vi "Calibration_Setting_UI.vi"(5 "Real Position Info":T5, 6 "CamGot?":bool, 7 "Cal Info Image":T1, 8 "error in (no error)":errorcluster, 9 "Cal Status In":bool, 10 "Root Path":path, 11 "Seq":string) -> (0 "error out":errorcluster, 2 "Calibration Done":bool, 3 "CalTemp":T1(plugin-control))   [LabVIEW 2019]
uses:
  <vilib>/vision/Image Controls.llb/IMAQ Image.ctl
  <vilib>/vision/Calibration.llb/Distortion Model.ctl
  <vilib>/vision/Calibration.llb/Distortion Model Types.ctl
  <vilib>/vision/Image Controls.llb/Vision Info Type2.ctl
  Controls/Parameter.ctl
  LLB/Commonly VI/Main Glb.vi
  <vilib>/vision/NI_Vision_Development_Module.lvlib
  LLB/Commonly VI.lvlib
panel:
  in  "Tab Control":enum32{"Page 1", "Page 2"}(tab)
  out "CalTemp 2":T1(plugin-control)
  out "Grid Descriptor 2":T2={"X Step"=1.0, "Y Step"=1.0, "Unit"=enum."Undefined"} {"Y Step" format="%.2f"; "X Step" format="%.2f"}
  in  "CamSelect":u16(ring) caption="相機" items=["cam0"]
  in  "Reset":bool
  in  "Camera Angle":enum32{"Parallel", "Perpendicular"}(radio)
  in  "Relative Position":T4={"Direction"=enum."Negative", "D"=100.0} {"D" min=1.0 step=1.0}
  in  "Reference Points":i32(listbox)
  in  "Use Real Position":bool
  in  "Grid Descriptor":cluster{"X Step":sgl, "Y Step":sgl, "Unit":T3}={"X Step"=10.0, "Y Step"=10.0, "Unit"=enum."Millimeter"}
  in  "Area Min":dbl=100.0
  in  "Area Max":dbl=1000.0
  in  "Run Cal":bool
  in  "CalExit":bool caption="Exit"
  in  "Done":bool
  in  "Snap":bool
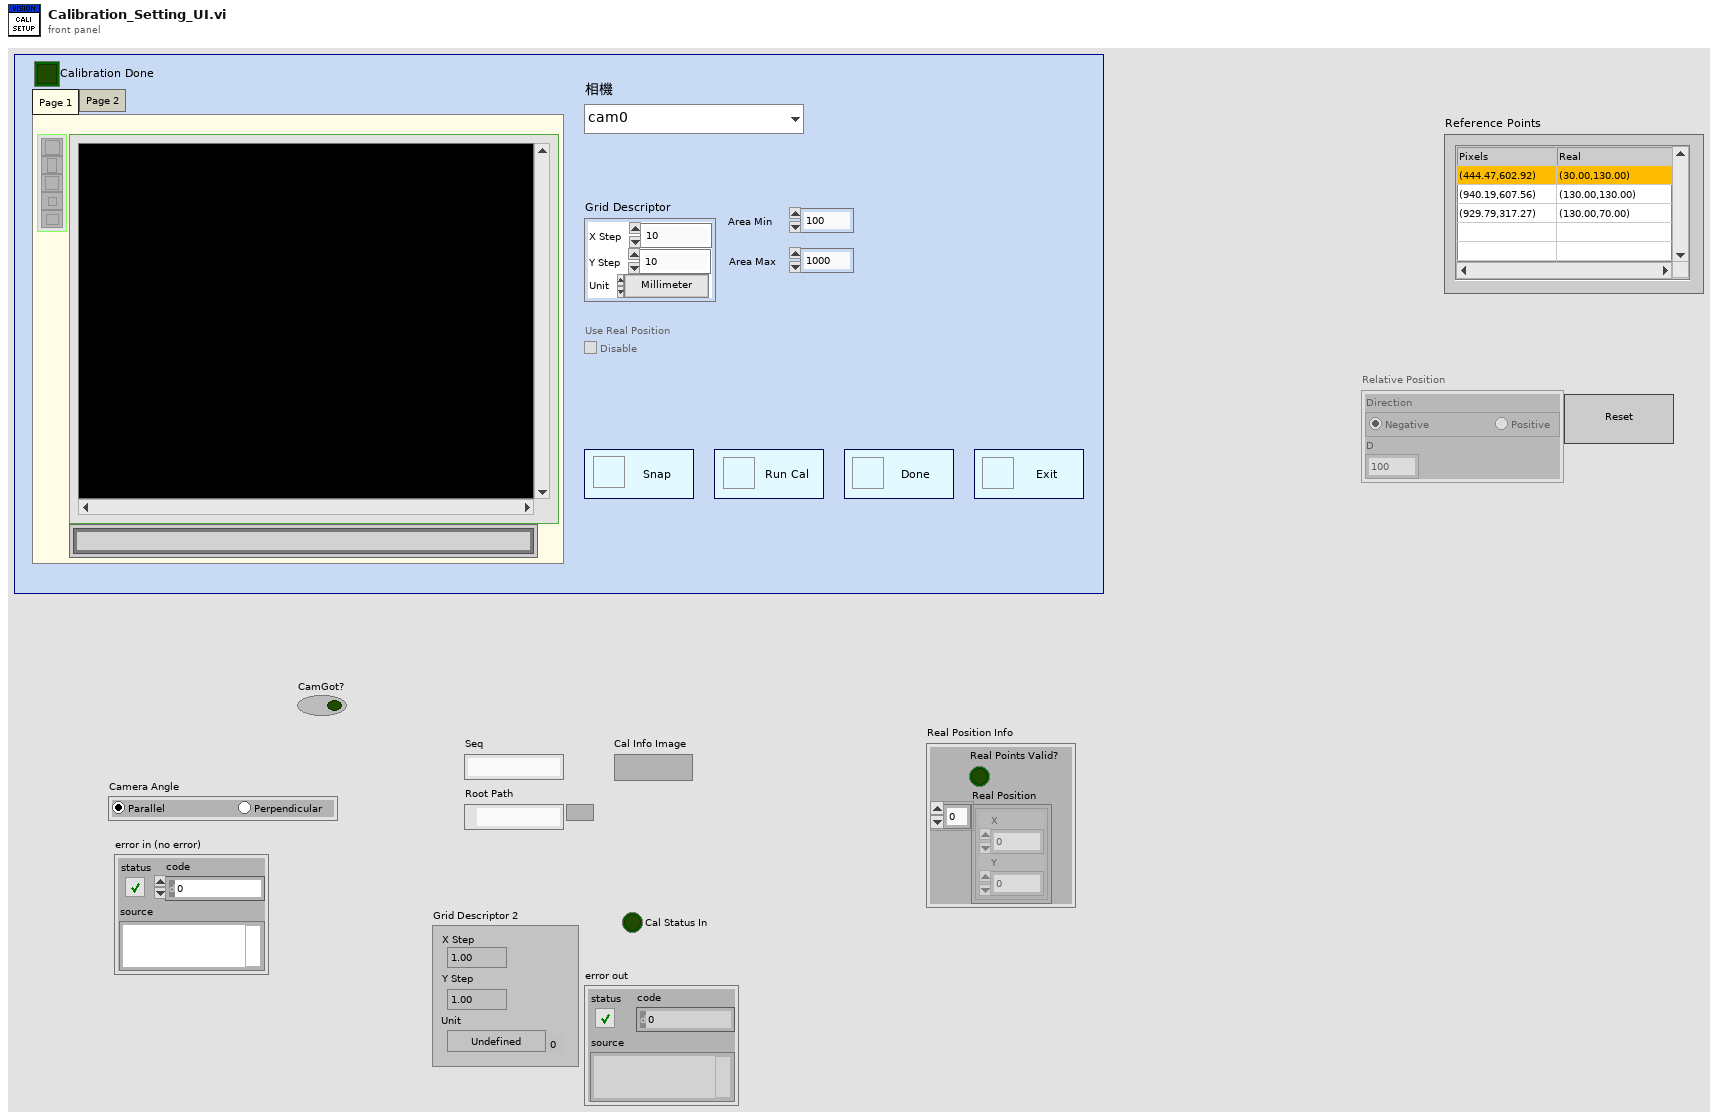
[diagram p1: front panel]
types:
  T1 = typedef "IMAQ Image.ctl" = refnum<image>
  T2 = typedef "Simple Grid Descriptor" = cluster{"X Step":sgl, "Y Step":sgl, "Unit":T3}
  T3 = typedef "Image Unit" = enum32{"Undefined", "Angström", "Micrometer", "Millimeter", "Centimeter", "Meter", "Kilometer", "Microinch", "Inch", "Feet", "Nautical miles", "Standard miles", "Steps"}
  T4 = cluster{"Direction":enum32{"Negative", "Positive"}, "D":dbl}
  T5 = cluster{"Real Points Valid?":bool, "Real Position":cluster{"X":dbl, "Y":dbl}[]}
  T6 = typedef "Image Type" = u32
  T7 = cluster{"Pixel":cluster{"X":dbl, "Y":dbl}[], "Real":cluster{"X":dbl, "Y":dbl}[]}
  T8 = enum16{"Init", "Grab", "Get All", "Close", "Set Camera"}
  T9 = enum8{"Enabled", "Disabled", "Disabled and Grayed Out"}
  T10 = typedef "Distortion Model.ctl" = cluster{"Distortion Model":T11, "Polynomial Model Setup":cluster{"Radial Coefficient":u32, "Tangential Coefficients ":bool}}
  T11 = typedef "Distortion Model Types.ctl" = i32
  T12 = typedef "Parameter.ctl" = enum16{"Initialize", "Write", "Read", "WriteAll", "Save", "Load"}
  T13 = typedef "IMAQdx.ctl" = refnum<k21>
  T14 = cluster{"Global Rectangle":i32[], "Contours":cluster{"Contour Type":u32, "ROI Type":u32, "Points":i32[]}[]}
  T15 = typedef "Calibration Reference Points.ctl" = cluster{"Pixel Coordinates":cluster{"X":dbl, "Y":dbl}[], "Real World Coordinates":cluster{"X":dbl, "Y":dbl}[], "Unit":T3, "Image Size":cluster{"X":u32, "Y":u32}}
  T16 = typedef "ROI Descriptor" = cluster{"Global Rectangle":i32[], "Contours":cluster{"ID":enum32{"External", "Internal"}, "Type":u32, "Coordinates":i32[]}[]}
  T17 = cluster{"Global Rectangle[0]":i32, "Global Rectangle[1]":i32, "Global Rectangle[2]":i32, "Global Rectangle[3]":i32}
  T18 = enum32{"invalid app kind", "Development System", "Run Time System", "Student Edition", "Embedded LabVIEW", "Evaluation", "Custom"}
  T19 = typedef "Vision Info Type2.ctl" = u32
  T20 = cluster{"histogram":u32[], "Minimal Value":sgl, "Maximal Value":sgl, "Starting Value":sgl, "Interval Width":sgl, "Mean Value":sgl, "Standard  Variation":sgl, "Area (pixels)":i32}
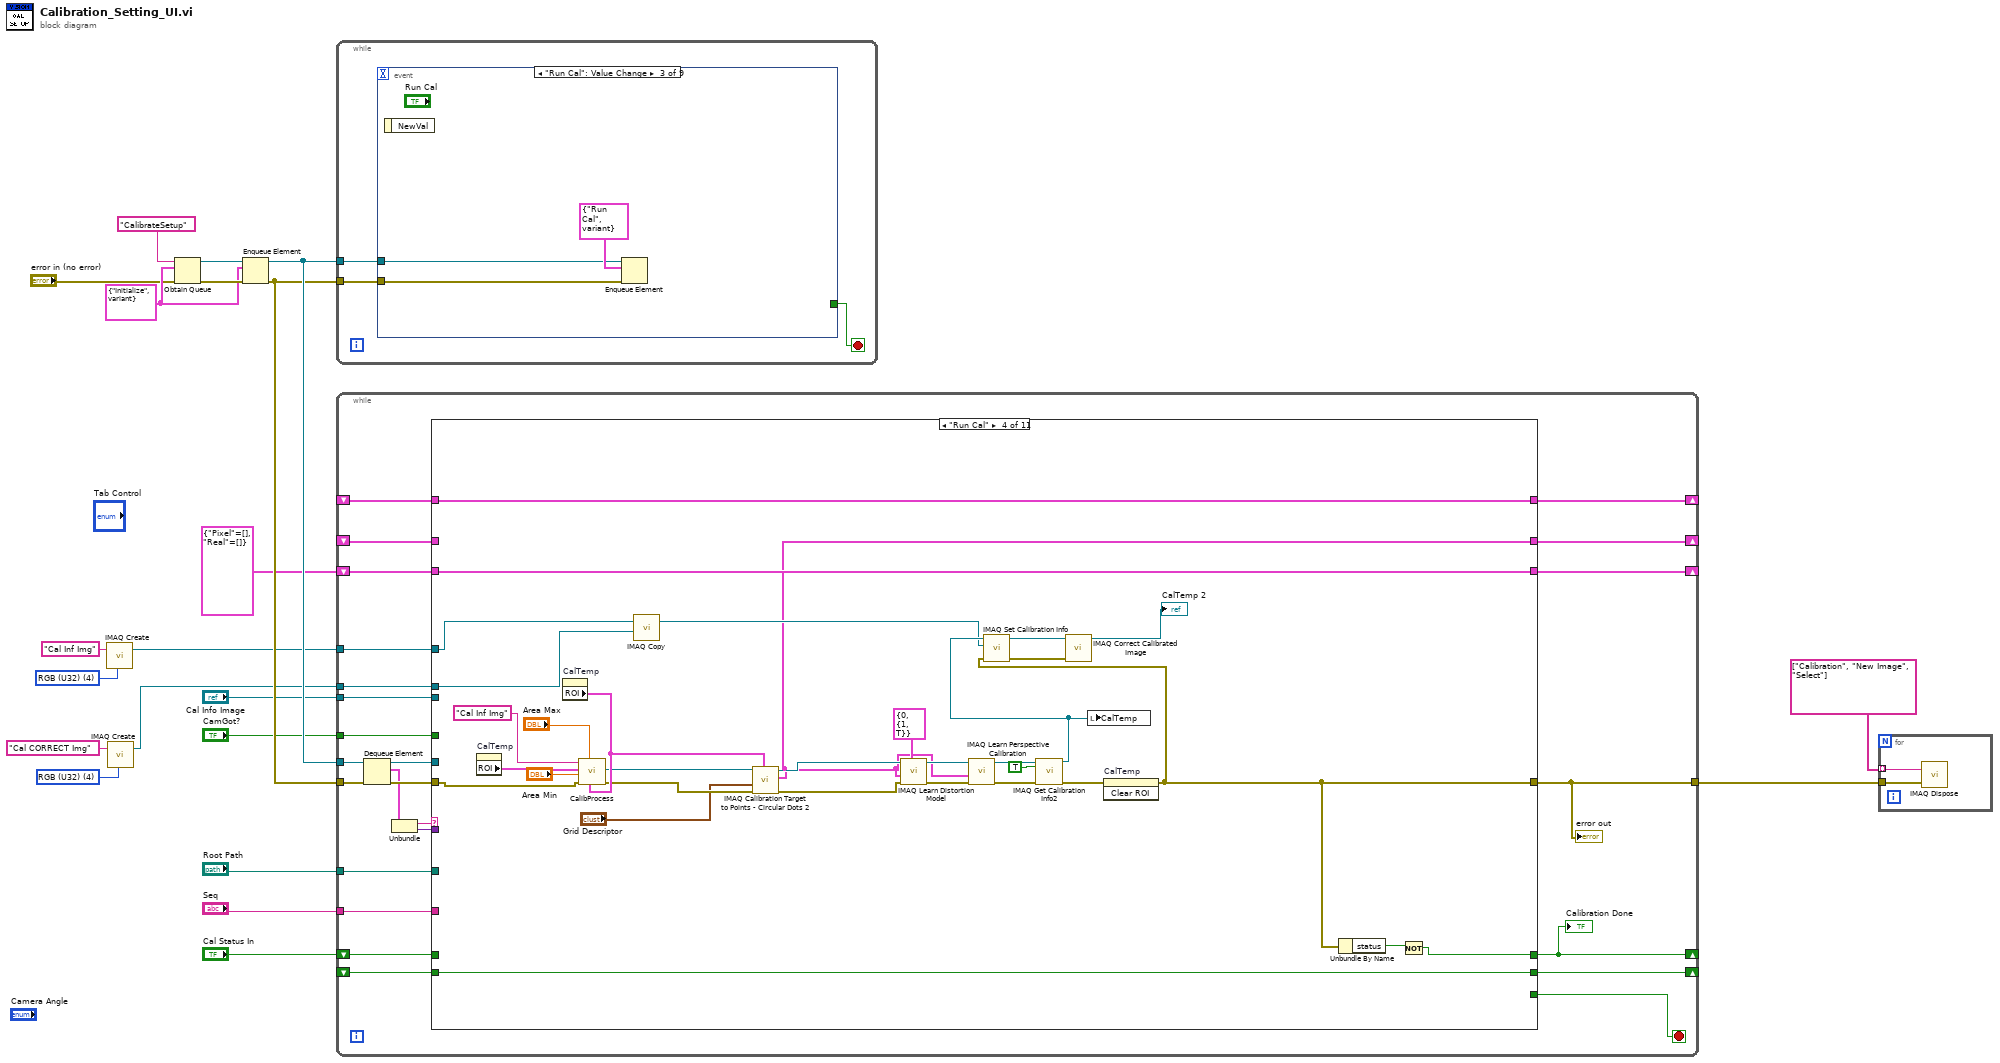
[diagram p0: block diagram]
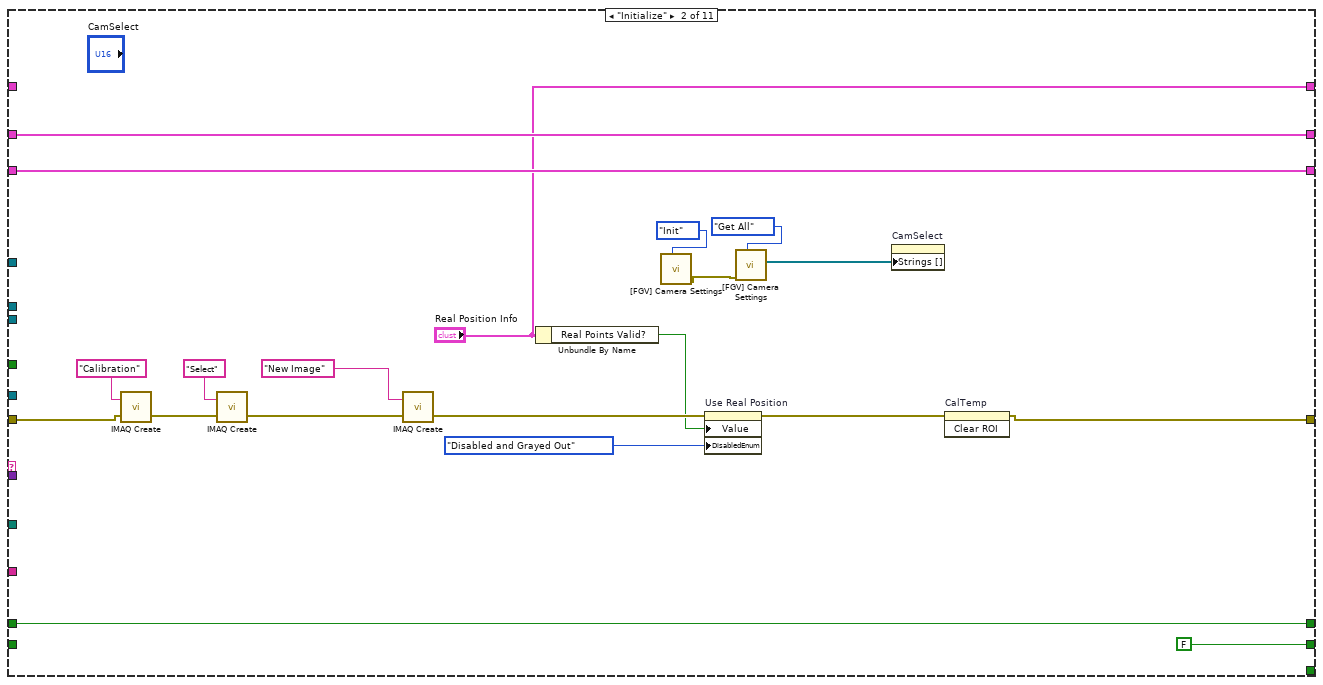
[diagram p3: hidden frame]
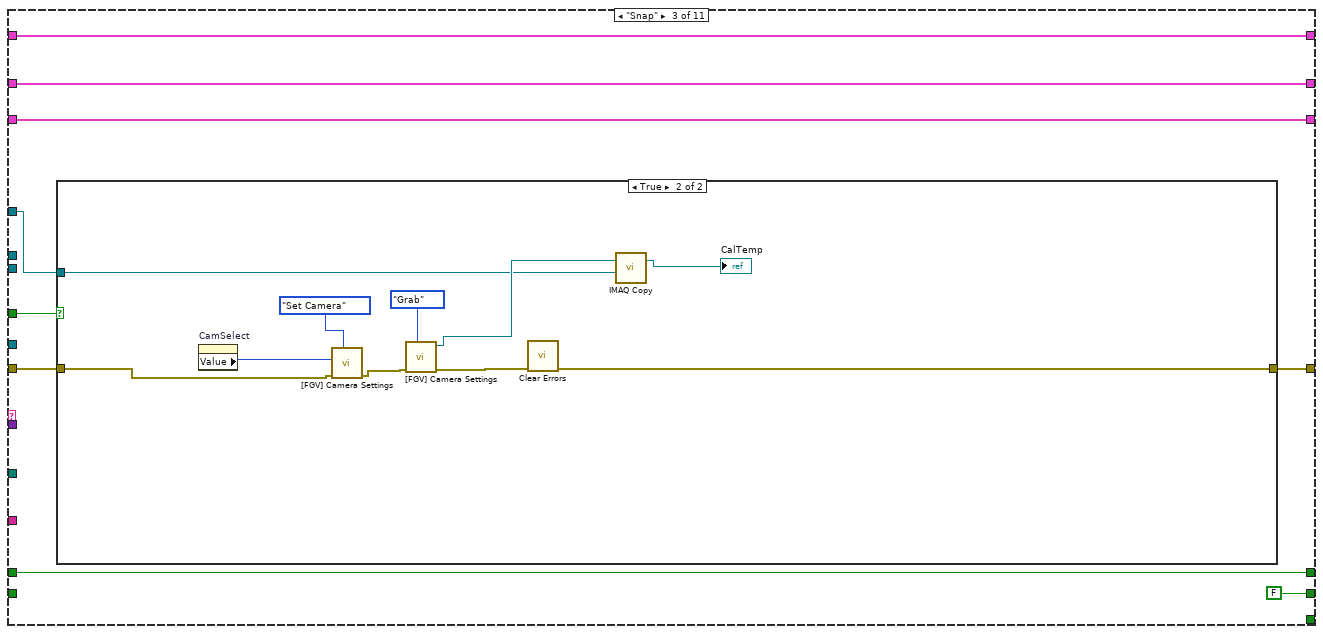
[diagram p4: hidden frame]
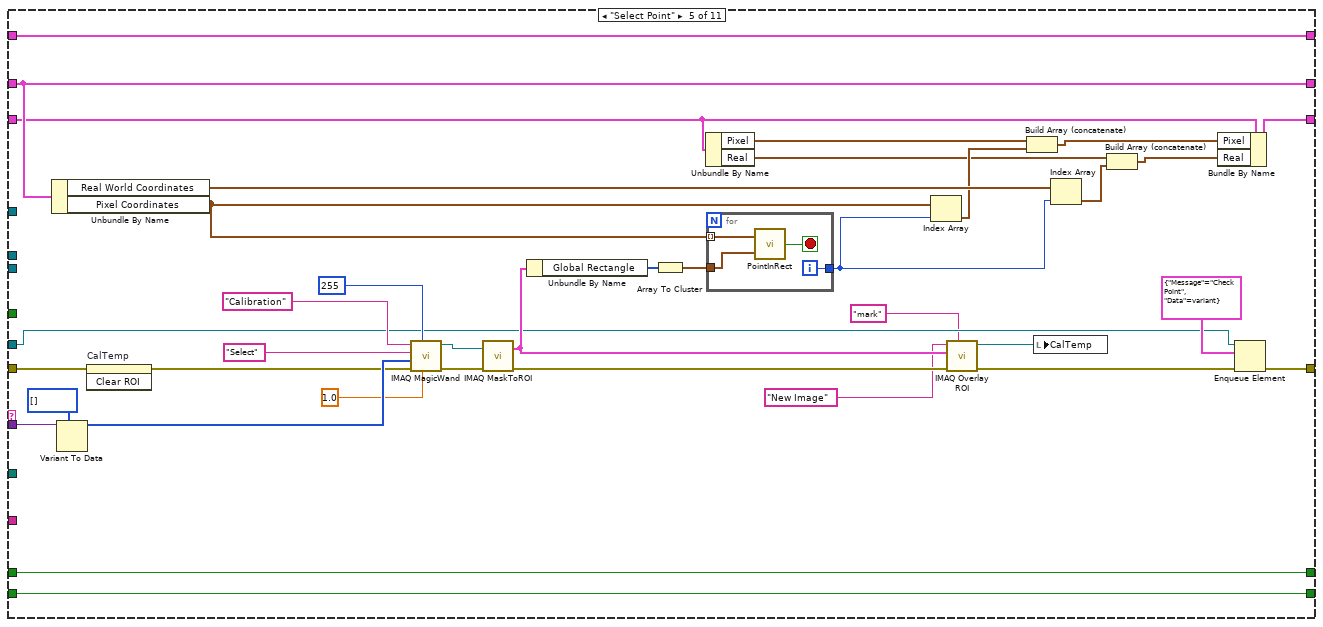
[diagram p6: hidden frame]
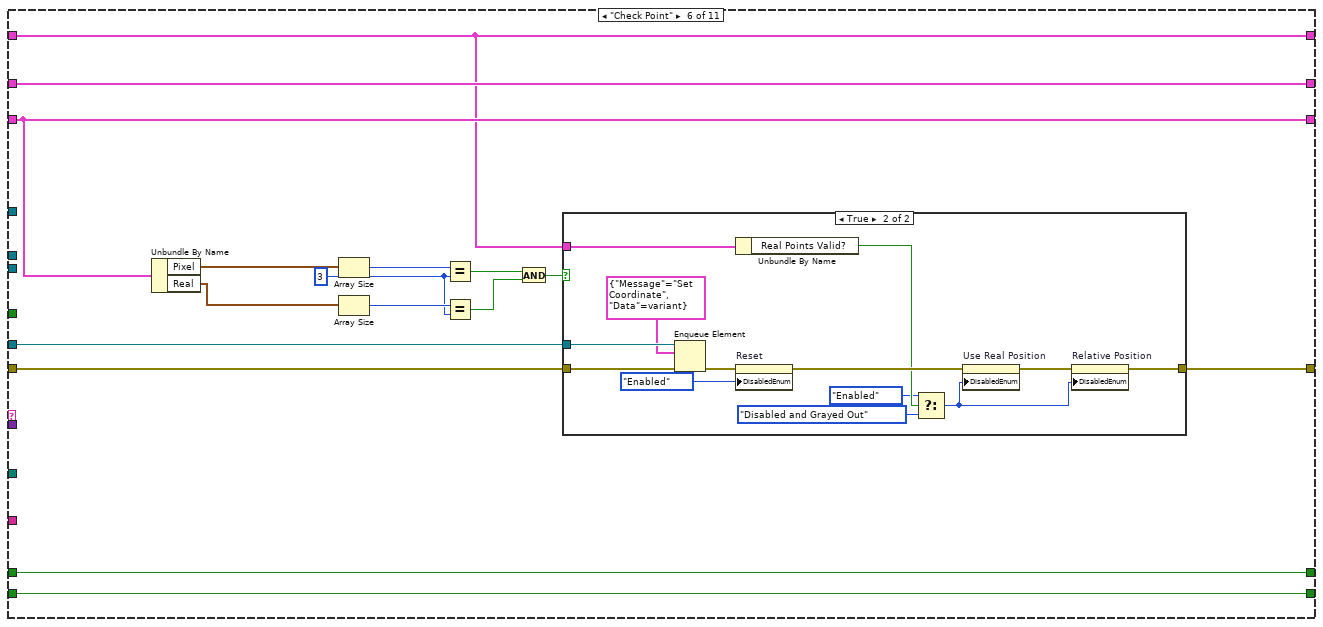
[diagram p7: hidden frame]
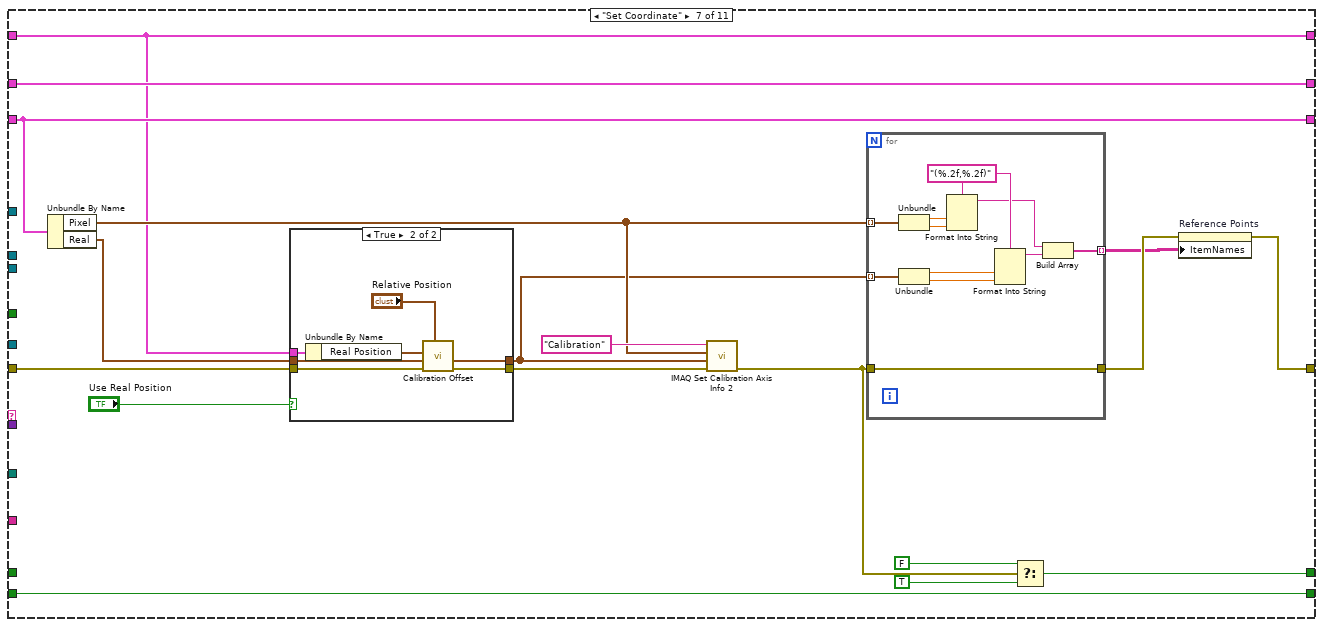
[diagram p9: hidden frame]
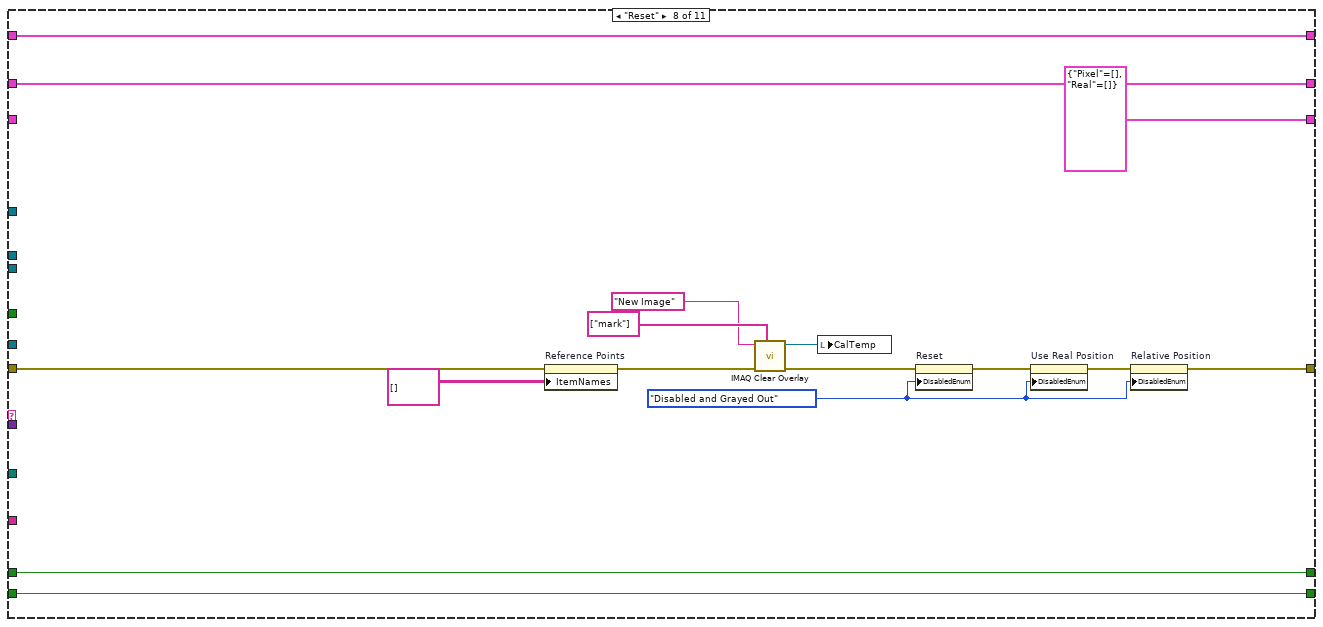
[diagram p11: hidden frame]
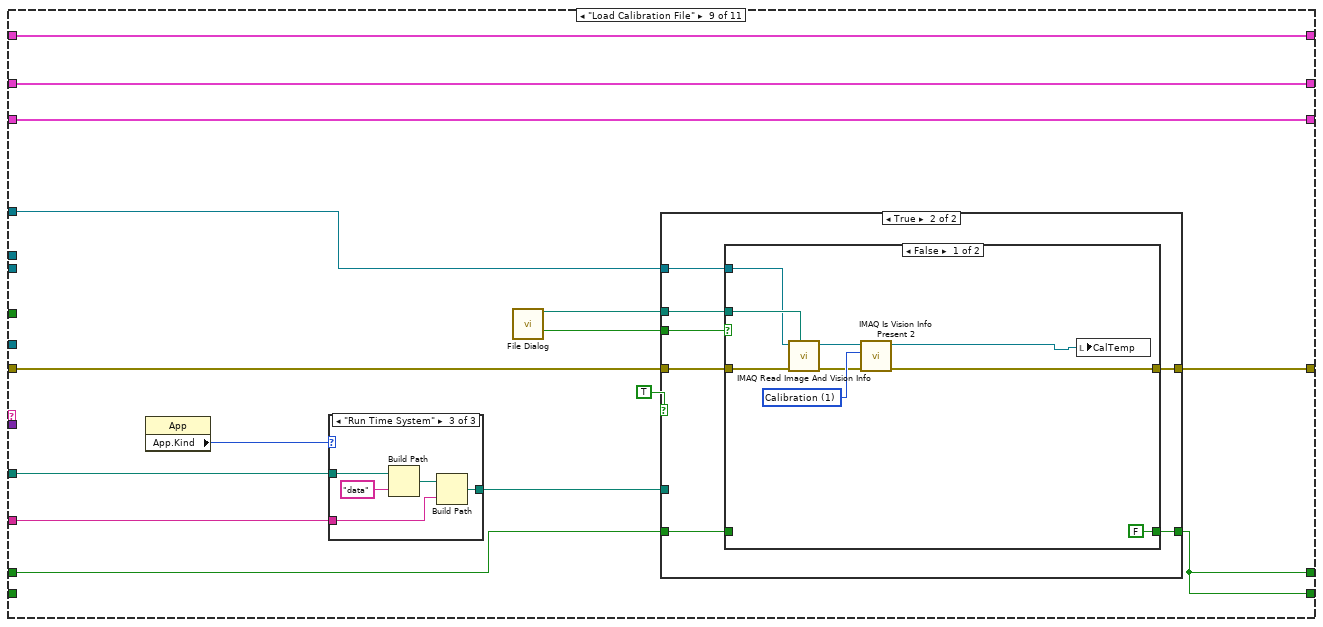
[diagram p12: hidden frame]
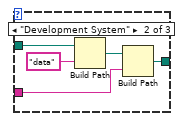
[diagram p14: hidden frame]
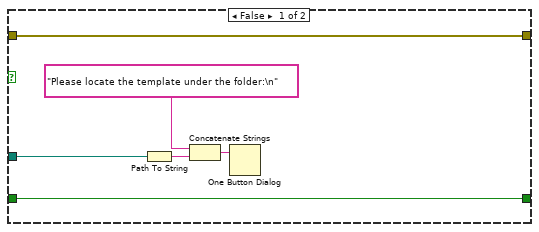
[diagram p15: hidden frame]
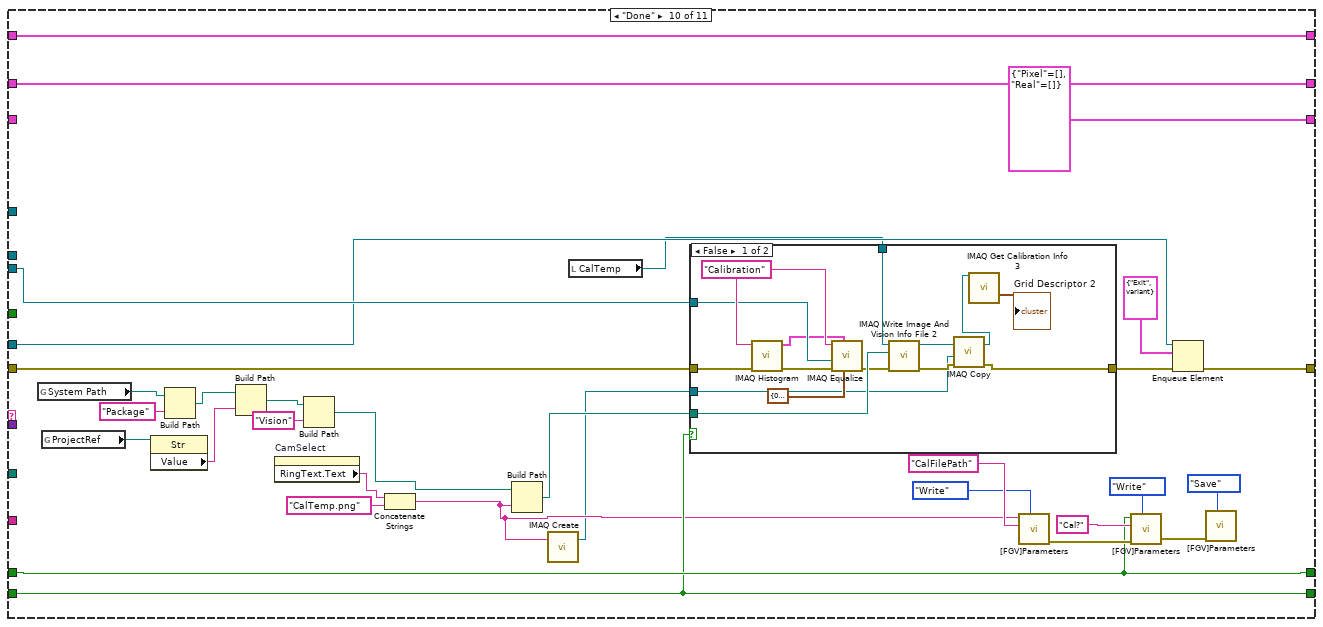
[diagram p17: hidden frame]
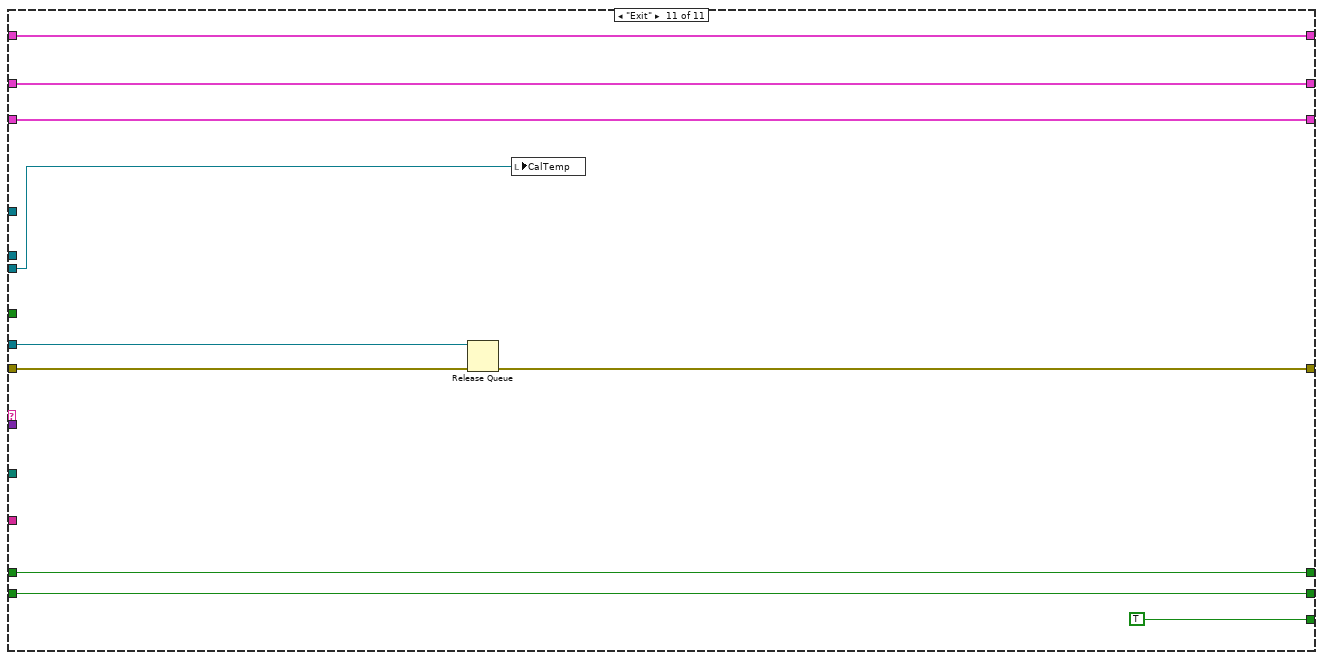
[diagram p19: hidden frame]
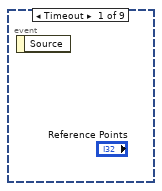
[diagram p20: hidden frame]
diagram:
  w3 = T6 4 items=["Grayscale (U8)", "Grayscale (I16)", "Grayscale (SGL)", "Complex (CSG)", "RGB (U32)", "HSL (U32)", "RGB (U64)", "Grayscale (U16)"] ("Image Type")
  w5 = T6 4 items=["Grayscale (U8)", "Grayscale (I16)", "Grayscale (SGL)", "Complex (CSG)", "RGB (U32)", "HSL (U32)", "RGB (U64)", "Grayscale (U16)"] ("Image Type")
  w16 = cluster{"Message":string, "Data":variant} {"Message"="Initialize", "Data"=variant}
  n1 = call "IMAQ Create"("Image Name"="Cal Inf Img", "Image Type"=w5) -> ("New Image"=w4:T1)  [unwired: 3 in, 1 out]
  n2 = call "IMAQ Create"("Image Name"="Cal CORRECT Img", "Image Type"=w3) -> ("New Image"=w1:T1)  [unwired: 3 in, 1 out]
  n3 = Obtain Queue(name (unnamed)="CalibrateSetup", element data type=w16, error in (no error)="error in (no error)") -> (queue out=w20:refnum<queue>, error out=w19:errorcluster)  [unwired: 2 in, 1 out]
  n4 = Enqueue Element(queue=w20, element=w16, error in (no error)=w19) -> (queue out=w18:refnum<queue>, error out=w17:errorcluster)  [unwired: 1 in, 1 out]
  n5 = while {
    tunnel: w18 -> [w24]
    tunnel: w17 -> [w23]
    stop <- w22 stop-if-true
    n6 = event shown="[2] \"Run Cal\": Value Change" {
      selector: _ -> [_ _ _ _ _ _ _ _ _]
      dyn-events: _ -> [_ _ _ _ _ _ _ _ _]
      timeout: _ -> [_ _ _ _ _ _ _ _ _]
      tunnel: w24 -> [_ w27 w29 w34 w43 w46 w48 w56 w59]
      tunnel: w23 -> [_ w26 w28 w33 w42 w45 w49 w55 w60]
      tunnel: [_ _ _ _ _ _ _ TRUE TRUE] -> w22
      event Timeout {
        n7 = event-data() -> ()  [unwired: 1 in, 1 out]
      }
      event "Snap": Value Change {
        n8 = event-data() -> ()  [unwired: 1 in, 1 out]
        n9 = Enqueue Element(queue=w27, element=cluster{"Message":string, "Data":variant} {"Message"="Snap", "Data"=variant}, error in (no error)=w26) -> ()  [unwired: 1 in, 3 out]
      }
      event "Run Cal": Value Change {
        n10 = event-data() -> ()  [unwired: 1 in, 1 out]
        n11 = Enqueue Element(queue=w29, element=cluster{"Message":string, "Data":variant} {"Message"="Run Cal", "Data"=variant}, error in (no error)=w28) -> ()  [unwired: 1 in, 3 out]
      }
      event "CalTemp": Mouse Up {
        w31 = i32[] [1] items=["No Event"=0, "Click Event"=1, "Draw Event"=2, "Size Event"=4, "Scroll Event"=5, "Double Click Event"=8] ("Which Events")
        n12 = event-data() -> ("CtlRef"=w36:refnum<vi>)  [unwired: 1 in]
        n13 = invoke class="ImageControl" method="Get Last Event"(reference=w36, "Which Events"=w31) -> ("Tool"=w35:i32, "Coordinates"=w32:i32[])  [unwired: 6 in, 6 out]
        n14 = case shown="2" w35 {
          tunnel: w34 -> [_ w41]
          tunnel: w33 -> [_ w40]
          tunnel: w32 -> [_ w38]
          frame 0, Default {
          }
          frame 2 {
            n15 = Bundle By Name(cluster=cluster{"Message":string, "Data":variant} {"Message"="Select Point", "Data"=variant}, "Data"=w38) -> (w37:cluster{"Message":string, "Data":variant})
            n16 = Enqueue Element(queue=w41, element=w37, error in (no error)=w40) -> ()  [unwired: 1 in, 3 out]
          }
        }
      }
      event "Reset": Value Change {
        n17 = event-data() -> ()  [unwired: 1 in, 1 out]
        n18 = Enqueue Element(queue=w43, element=cluster{"Message":string, "Data":variant} {"Message"="Reset", "Data"=variant}, error in (no error)=w42) -> ()  [unwired: 1 in, 3 out]
      }
      event "Use Real Position", "Relative Position": Value Change {
        n19 = event-data() -> ()  [unwired: 1 in, 6 out]
        n20 = Enqueue Element(queue=w46, element=cluster{"Message":string, "Data":variant} {"Message"="Set Coordinate", "Data"=variant}, error in (no error)=w45) -> ()  [unwired: 1 in, 3 out]
      }
      event Menu Selection (User) {
        n21 = event-data() -> ("ItemTag"=w50:string)  [unwired: 1 in]
        n22 = case shown="\"Load Calibration File\"" w50 {
          tunnel: w49 -> [_ w52]
          tunnel: w48 -> [_ w51]
          frame Default {
          }
          frame "Load Calibration File" {
            n23 = Enqueue Element(queue=w51, element=cluster{"Message":string, "Data":variant} {"Message"="Load Calibration File", "Data"=variant}, error in (no error)=w52) -> ()  [unwired: 1 in, 3 out]
          }
        }
      }
      event "Done": Value Change {
        n24 = event-data() -> ()  [unwired: 1 in, 1 out]
        n25 = Enqueue Element(queue=w56, element=cluster{"Message":string, "Data":variant} {"Message"="Done", "Data"=variant}, error in (no error)=w55) -> ()  [unwired: 1 in, 3 out]
      }
      event "CalExit": Value Change {
        n26 = event-data() -> ()  [unwired: 1 in, 1 out]
        n27 = Enqueue Element(queue=w59, element=cluster{"Message":string, "Data":variant} {"Message"="Exit", "Data"=variant}, error in (no error)=w60) -> ()  [unwired: 1 in, 3 out]
      }
    }
  }
  n28 = while {
    tunnel: w17 -> [w86]
    tunnel: w18 -> [w85]
    shift-right: [w80] -> _
    shift-left: _ -> [w79]
    shift-right: [w76] -> _
    shift-left: T7 {"Pixel"=[], "Real"=[]} ("Select Point") -> [w78]
    shift-right: [w75] -> _
    shift-left: _ -> [w74]
    tunnel: "Root Path" -> [w73]
    tunnel: "Seq" -> [w72]
    tunnel: "Cal Info Image" -> [w71]
    shift-right: [w69] -> _
    shift-left: "Cal Status In" -> [w70]
    shift-right: [w68] -> _
    shift-left: _ -> [w67]
    tunnel: "CamGot?" -> [w65]
    tunnel: [w64] -> w7
    tunnel: w4 -> [w63]
    tunnel: w1 -> [w62]
    stop <- w66 stop-if-true
    n29 = Dequeue Element(queue=w85, error in (no error)=w86) -> (queue out=w83:refnum<queue>, element=w82:cluster{"Message":string, "Data":variant}, error out=w84:errorcluster)  [unwired: 1 in, 1 out]
    n30 = Unbundle(w82) -> ("Message"=w81:string, "Data"=w77:variant)
    n31 = case shown="\"Run Cal\"" w81 {
      tunnel: w84 -> [w87 w111 w120 w151 w192 w217 w238 w286 w296 w367 w392]
      tunnel: w83 -> [_ _ _ _ w169 w218 _ _ _ w354 w393]
      tunnel: [w92 w110 w121 w135 w197 w221 w252 w288 w303 w370 w395] -> w80
      tunnel: w79 -> [w92 w110 w121 _ w197 w221 w252 w288 w303 w370 w395]
      tunnel: w78 -> [w91 w107 w119 w157 w174 w210 w251 _ w302 _ w394]
      tunnel: [w91 w107 w119 w157 w175 w210 w251 T7 {"Pixel"=[], "Real"=[]} ("Select Point") w302 T7 {"Pixel"=[], "Real"=[]} ("Select Point") w394] -> w76
      tunnel: w77 -> [_ _ _ _ w196 _ _ _ _ _ _]
      tunnel: [_ _ _ _ _ _ _ _ _ _ TRUE] -> w66
      tunnel: [w90 "Real Position Info" w118 w156 w172 w207 w237 w289 w304 w368 w396] -> w75
      tunnel: w74 -> [w90 _ w118 w156 w172 w207 w237 w289 w304 w368 w396]
      tunnel: w73 -> [_ _ _ _ _ _ _ _ w298 _ _]
      tunnel: w72 -> [_ _ _ _ _ _ _ _ w297 _ _]
      tunnel: w71 -> [_ _ _ _ _ _ _ _ _ w366 w387]
      tunnel: w70 -> [w89 w102 w117 _ w167 w209 _ w280 w295 w359 w390]
      tunnel: [w89 w102 w117 w148 w167 w209 w240 w280 w294 w359 w390] -> w69
      tunnel: [w88 FALSE ("Cal Status In") FALSE ("Cal Status In") w155 w166 w208 w241 w279 w294 w358 w389] -> w68
      tunnel: w67 -> [w88 _ _ w155 w166 w208 w241 w279 _ w358 w389]
      tunnel: w65 -> [_ _ w115 _ _ _ _ _ _ _ _]
      tunnel: [w87 w97 w114 w141 w165 w206 w236 w274 w293 w355 w388] -> w64
      tunnel: w63 -> [_ _ w113 w145 _ _ _ _ w290 _ _]
      tunnel: w62 -> [_ _ _ w146 _ _ _ _ _ _ _]
      frame Default {
      }
      frame "Initialize" {
        n32 = call "IMAQ Create"("Image Name"="Calibration", "error in (no error)"=w111) -> ("error out"=w108:errorcluster)  [unwired: 3 in, 1 out]
        n33 = call "IMAQ Create"("Image Name"="Select", "error in (no error)"=w108) -> ("error out"=w104:errorcluster)  [unwired: 3 in, 1 out]
        n34 = call "IMAQ Create"("Image Name"="New Image", "error in (no error)"=w104) -> ("error out"=w103:errorcluster)  [unwired: 3 in, 1 out]
        n35 = Unbundle By Name("Real Position Info") -> ("Real Points Valid?"=w100:bool)
        n36 = call "[FGV] Camera Settings.vi"("Action"=T8."Init") -> ("error out"=w93:errorcluster)  [unwired: 8 in, 2 out]
        n37 = property on="Use Real Position" class="Bool (strict)"(error in=w103, "Value"=w100, "DisabledEnum"=T9."Disabled and Grayed Out" ("Disabled")) -> (error out=w106:errorcluster)  [unwired: 1 in, 1 out]
        n38 = call "[FGV] Camera Settings.vi"("Action"=T8."Get All", "error in (no error)"=w93) -> ("Camera Interface Name"=w95:T13[])  [unwired: 7 in, 2 out]
        n39 = property on="CamSelect" class="Ring (strict)"("Strings []"=w95) -> ()  [unwired: 2 in, 2 out]
        n40 = invoke on="CalTemp" class="ImageControl" method="Clear ROI"(error in=w106) -> (error out=w97:errorcluster)  [unwired: 2 in, 2 out]
      }
      frame "Snap" {
        n41 = case shown="True" w115 {
          tunnel: w120 -> [w122 w123]
          tunnel: [w122 w130] -> w114
          tunnel: w113 -> [_ w128]
          frame False {
          }
          frame True {
            n42 = property on="CamSelect" class="Ring (strict)"() -> ("Value"=w125:u16)  [unwired: 2 in, 2 out]
            n43 = call "[FGV] Camera Settings.vi"("Action"=T8."Set Camera", "error in (no error)"=w123, "Value"=w125) -> ("error out"=w124:errorcluster)  [unwired: 6 in, 2 out]
            n44 = call "[FGV] Camera Settings.vi"("Action"=T8."Grab", "error in (no error)"=w124) -> ("error out"=w132:errorcluster, "Image Out"=w129:T1)  [unwired: 7 in, 1 out]
            n45 = call <vilib>:"Clear Errors.vi"("error in (no error)"=w132) -> ("error out"=w130:errorcluster)  [unwired: 5 in, 1 out]
            n46 = call "IMAQ Copy"("Image Dst"=w128, "Image Src"=w129) -> ("Image Dst Out"=→"CalTemp":T1)  [unwired: 4 in, 1 out]
          }
        }
      }
      frame "Run Cal" {
        n47 = property on="CalTemp" class="ImageControl"() -> ("ROI"=w154:T14)  [unwired: 2 in, 2 out]
        n48 = property on="CalTemp" class="ImageControl"() -> ("ROI"=w139:T14)  [unwired: 2 in, 2 out]
        n49 = call "CalibProcess.vi"("ROI Descriptor"=w139, "Area Max"="Area Max", "error in (no error)"=w151, "Area Min"="Area Min", "ROI"=w154, "Refnum in"="Cal Inf Img" ("Image Name")) -> ("error out"=w137:errorcluster, "Image Dst Out"=w133:T1)  [unwired: 3 in, 1 out]
        n50 = call "IMAQ Copy"("Image Dst"=w146, "Image Src"=w145) -> ("Image Dst Out"=w142:T1)  [unwired: 4 in, 1 out]
        n51 = call "IMAQ Calibration Target to Points - Circular Dots 2"("ROI Descriptor"=w139, "error in (no error)"=w137, "Grid Descriptor"="Grid Descriptor", "Target Image"=w133) -> ("error out"=w136:errorcluster, "Reference Points"=w135:T15, "Target Image (dup)"=w138:T1)  [unwired: 5 in]
        n52 = call "IMAQ Learn Distortion Model"("Distortion Model Setup"=T10 {"Distortion Model"=0, "Polynomial Model Setup"={"Radial Coefficient"=1, "Tangential Coefficients "=TRUE}}, "error in (no error)"=w136, "Reference Points"=w135, "Calibration Template Image"=w138) -> ("error out"=w160:errorcluster, "Calibration Template Image Out"=w163:T1)  [unwired: 2 in, 4 out]
        n53 = call "IMAQ Learn Perspective Calibration"("error in (no error)"=w160, "Reference Points"=w135, "Calibration Template Image"=w163) -> ("error out"=w159:errorcluster, "Calibration Template Image Out"=w162:T1)  [unwired: 1 in, 6 out]
        n54 = call "IMAQ Get Calibration Info2"("Calibration Template Image"=w162, "Return Error Information (False)"=TRUE, "error in (no error)"=w159) -> ("Calibration Template Image (duplicate)"=w143:T1, "error out"=w158:errorcluster)  [unwired: 11 out]
        n55 = local write "CalTemp"(w143) -> ()
        n56 = invoke on="CalTemp" class="ImageControl" method="Clear ROI"(error in=w158) -> (error out=w141:errorcluster)  [unwired: 2 in, 2 out]
        n57 = call "IMAQ Set Calibration Info"("error in (no error)"=w141, "Image Dst"=w142, "Image Src"=w143) -> ("error out"=w140:errorcluster, "Calibrated Image"=w144:T1)  [unwired: 1 in, 6 out]
        n58 = call "IMAQ Correct Calibrated Image"("error in (no error)"=w140, "Image Src"=w144) -> ("Corrected Image"=→"CalTemp 2":T1)  [unwired: 8 in, 1 out]
        n59 = Unbundle By Name(w141) -> ("status"=w149:bool)
        n60 = Not(x=w149) -> (.not. x?=w148:bool)
      }
      frame "Select Point" {
        n61 = Unbundle By Name(w197) -> ("Real World Coordinates"=w183:cluster{"X":dbl, "Y":dbl}[], "Pixel Coordinates"=w200:cluster{"X":dbl, "Y":dbl}[])
        n62 = Variant To Data(type=i32[] [], Variant=w196) -> (data=w195:i32[])  [unwired: 1 in, 1 out]
        n63 = invoke on="CalTemp" class="ImageControl" method="Clear ROI"(error in=w192) -> (error out=w191:errorcluster)  [unwired: 2 in, 2 out]
        n64 = call "IMAQ MagicWand"("Tolerance"=sgl 1.0, "Fill Value"=u8 255, "error in (no error)"=w191, "Hot spot (x,y)"=w195, "Image Dst"="Select" ("Image Name"), "Image Src"="Calibration" ("Image Name")) -> ("error out"=w201:errorcluster, "Image Dst Out"=w188:T1)  [unwired: 4 in]
        n65 = call "IMAQ MaskToROI"("Image"=w188, "error in (no error)"=w201) -> ("ROI Descriptor"=w186:T16, "error out"=w184:errorcluster)  [unwired: 5 in, 1 out]
        n66 = Unbundle By Name(w186) -> ("Global Rectangle"=w198:i32[])
        n67 = Array To Cluster(array=w198) -> (cluster=w199:T17)
        n68 = Unbundle By Name(w174) -> ("Pixel"=w181:cluster{"X":dbl, "Y":dbl}[], "Real"=w178:cluster{"X":dbl, "Y":dbl}[])
        n69 = for {
          tunnel: w199 -> [w205]
          tunnel: w200 -> [w204] mode=indexing
          tunnel: [w202] -> w182
          i -> [w202]
          stop <- w203 stop-if-true
          n70 = call <vilib>:"PointInRect.vi"("rect"=w205, "point"=w204) -> ("pt in rect"=w203:bool)
        }
        n71 = Index Array(array=w200, index=w182) -> (element=w180:cluster{"X":dbl, "Y":dbl})
        n72 = call "IMAQ Overlay ROI"("Group"="mark", "error in (no error)"=w184, "ROI Descriptor"=w186, "Image"="New Image" ("Image Name")) -> ("error out"=w170:errorcluster, "Image Out"=w185:T1)  [unwired: 6 in]
        n73 = Build Array (concatenate)(w181, w180) -> (w179:cluster{"X":dbl, "Y":dbl}[])
        n74 = local write "CalTemp"(w185) -> ()
        n75 = Index Array(array=w183, index=w182) -> (element=w177:cluster{"X":dbl, "Y":dbl})
        n76 = Build Array (concatenate)(w178, w177) -> (w176:cluster{"X":dbl, "Y":dbl}[])
        n77 = Bundle By Name(cluster=w174, "Pixel"=w179, "Real"=w176) -> (w175:T7)
        n78 = Enqueue Element(queue=w169, element=cluster{"Message":string, "Data":variant} {"Message"="Check Point", "Data"=variant}, error in (no error)=w170) -> (error out=w165:errorcluster)  [unwired: 1 in, 2 out]
      }
      frame "Check Point" {
        w213 = 3 ("y")
        n79 = Unbundle By Name(w210) -> ("Pixel"=w216:cluster{"X":dbl, "Y":dbl}[], "Real"=w214:cluster{"X":dbl, "Y":dbl}[])
        n80 = Array Size(array=w216) -> (size(s)=w220:i32)
        n81 = Array Size(array=w214) -> (size(s)=w215:i32)
        n82 = Equal?(x=w220, y=w213) -> (x = y?=w219:bool)
        n83 = Equal?(x=w215, y=w213) -> (x = y?=w211:bool)
        n84 = And(x=w219, y=w211) -> (x .and. y?=w212:bool)
        n85 = case shown="True" w212 {
          tunnel: w218 -> [_ w235]
          tunnel: w217 -> [w222 w234]
          tunnel: w207 -> [_ w229]
          tunnel: [w222 w223] -> w206
          frame False {
          }
          frame True {
            n86 = Enqueue Element(queue=w235, element=cluster{"Message":string, "Data":variant} {"Message"="Set Coordinate", "Data"=variant}, error in (no error)=w234) -> (error out=w232:errorcluster)  [unwired: 1 in, 2 out]
            n87 = Unbundle By Name(w229) -> ("Real Points Valid?"=w227:bool)
            n88 = property on="Reset" class="Bool"(error in=w232, "DisabledEnum"=T9."Enabled" ("Disabled")) -> (error out=w231:errorcluster)  [unwired: 1 in, 1 out]
            n89 = Select(t=T9."Enabled" ("Disabled"), s=w227, f=T9."Disabled and Grayed Out") -> (s? t:f=w225:T9)
            n90 = property on="Use Real Position" class="Bool (strict)"(error in=w231, "DisabledEnum"=w225) -> (error out=w230:errorcluster)  [unwired: 1 in, 1 out]
            n91 = property on="Relative Position" class="Clust (strict)"(error in=w230, "DisabledEnum"=w225) -> (error out=w223:errorcluster)  [unwired: 1 in, 1 out]
          }
        }
      }
      frame "Set Coordinate" {
        n92 = Unbundle By Name(w251) -> ("Pixel"=w248:cluster{"X":dbl, "Y":dbl}[], "Real"=w249:cluster{"X":dbl, "Y":dbl}[])
        n93 = case shown="True" "Use Real Position" {
          tunnel: w249 -> [w266 w273]
          tunnel: [w266 w272] -> w247
          tunnel: [w265 w271] -> w239
          tunnel: w238 -> [w265 w270]
          tunnel: w237 -> [_ w269]
          frame False {
          }
          frame True {
            n94 = Unbundle By Name(w269) -> ("Real Position"=w267:cluster{"X":dbl, "Y":dbl}[])
            n95 = call "Calibration Offset.vi"("Relative Position"="Relative Position", "error in (no error)"=w270, "Calibraion Position In"=w273, "Real Position"=w267) -> ("error out"=w271:errorcluster, "Calibraion Position Out"=w272:cluster{"X":dbl, "Y":dbl}[])  [unwired: 6 in]
          }
        }
        n96 = call-poly "IMAQ Set Calibration Axis Info 2"("error in (no error)"=w239, "Real World Coordinates"=w247, "Pixel Coordinates"=w248, "Calibration Template Image In"="Calibration" ("Image Name")) -> ("error out"=w244:errorcluster)  [unwired: 6 in, 1 out]
        n97 = for {
          tunnel: w244 -> [w254]
          tunnel: w248 -> [w263] mode=indexing
          tunnel: w247 -> [w264] mode=indexing
          tunnel: [w255] -> w245 mode=indexing
          tunnel: [w254] -> w246
          w258 = "(%.2f,%.2f)" ("format string")
          n98 = Unbundle(w263) -> ("X"=w261:dbl, "Y"=w262:dbl)
          n99 = Unbundle(w264) -> ("X"=w259:dbl, "Y"=w260:dbl)
          n100 = Format Into String(format string=w258, w261, w262) -> (resulting string=w257:string)  [unwired: 2 in, 1 out]
          n101 = Format Into String(format string=w258, w259, w260) -> (resulting string=w256:string)  [unwired: 2 in, 1 out]
          n102 = Build Array(w257, w256) -> (w255:string[])
        }
        n103 = Select(t=FALSE, s=w244, f=TRUE) -> (s? t:f=w240:bool)
        n104 = property on="Reference Points" class="MCListbox (strict)"(error in=w246, "ItemNames"=w245) -> (error out=w236:errorcluster)  [unwired: 1 in, 1 out]
      }
      frame "Reset" {
        w275 = T9."Disabled and Grayed Out" ("Disabled")
        n105 = property on="Reference Points" class="MCListbox (strict)"(error in=w286, "ItemNames"=string[][] [] ("Item Names")) -> (error out=w282:errorcluster)  [unwired: 1 in, 1 out]
        n106 = call "IMAQ Clear Overlay"("Groups"=string[] ["mark"], "error in (no error)"=w282, "Image"="New Image" ("Image Name")) -> ("error out"=w277:errorcluster, "Image Out"=w281:T1)  [unwired: 7 in]
        n107 = local write "CalTemp"(w281) -> ()
        n108 = property on="Reset" class="Bool"(error in=w277, "DisabledEnum"=w275) -> (error out=w278:errorcluster)  [unwired: 1 in, 1 out]
        n109 = property on="Use Real Position" class="Bool (strict)"(error in=w278, "DisabledEnum"=w275) -> (error out=w276:errorcluster)  [unwired: 1 in, 1 out]
        n110 = property on="Relative Position" class="Clust (strict)"(error in=w276, "DisabledEnum"=w275) -> (error out=w274:errorcluster)  [unwired: 1 in, 1 out]
      }
      frame "Load Calibration File" {
        n111 = property class="App"() -> ("App.Kind"=w299:T18)  [unwired: 2 in, 2 out]
        n112 = case shown="\"Run Time System\"" w299 {
          tunnel: w298 -> [_ w309 w314]
          tunnel: w297 -> [_ w306 w311]
          tunnel: [_ w305 w310] -> w291
          frame "invalid app kind", Default {
          }
          frame "Development System" {
            n113 = Build Path(base path=w309, name or relative path="data") -> (appended path=w307:path)
            n114 = Build Path(base path=w307, name or relative path=w306) -> (appended path=w305:path)
          }
          frame "Run Time System" {
            n115 = Build Path(base path=w314, name or relative path="data") -> (appended path=w312:path)
            n116 = Build Path(base path=w312, name or relative path=w311) -> (appended path=w310:path)
          }
        }
        n117 = call "File Dialog"() -> ("selected path"=w300:path, "cancelled"=w301:bool)  [unwired: 12 in, 2 out]
        n118 = case shown="True" TRUE {
          tunnel: [w319 w327] -> w293
          tunnel: w296 -> [w319 w326]
          tunnel: w295 -> [w320 w325]
          tunnel: [w320 w324] -> w294
          tunnel: w301 -> [_ w323]
          tunnel: w290 -> [_ w322]
          tunnel: w300 -> [_ w321]
          tunnel: w291 -> [w317 _]
          frame False {
            n119 = Path To String(path=w317) -> (string=w316:string)
            n120 = Concatenate Strings("Please locate the template under the folder:\n" ("message"), w316) -> (w315:string)
            n121 = One Button Dialog(message=w315) -> ()  [unwired: 1 in, 1 out]
          }
          frame True {
            n122 = case shown="False" w323 {
              tunnel: [w331 w337] -> w327
              tunnel: w326 -> [w336 w337]
              tunnel: w325 -> [_ w338]
              tunnel: [FALSE ("Cal Status In") w338] -> w324
              tunnel: w321 -> [w332 _]
              tunnel: w322 -> [w330 _]
              frame False {
                w335 = T19 1 items=["Any", "Calibration", "Overlay", "Grayscale Template", "Color Template", "Geometric Template", "Custom Data", "Golden Template", "Geometric Template 2", "Contour Data", "Camera Model", "Pyramid Grayvalue Template", "Pyramid Gradient Template"] ("Vision Info")
                n123 = call "IMAQ Read Image And Vision Info"("File Path"=w332, "error in (no error)"=w336, "Image"=w330) -> ("error out"=w334:errorcluster, "Image Out"=w333:T1)  [unwired: 6 in, 1 out]
                n124 = call "IMAQ Is Vision Info Present 2"("error in (no error)"=w334, "Vision Info"=w335, "Image"=w333) -> ("error out"=w331:errorcluster, "Image (duplicate)"=w329:T1)  [unwired: 6 in, 1 out]
                n125 = local write "CalTemp"(w329) -> ()
              }
              frame True {
              }
            }
          }
        }
      }
      frame "Done" {
        n126 = global read "Main Glb.vi" "System Path"() -> (w341:path)
        n127 = global read "Main Glb.vi" "ProjectRef"() -> (w353:refnum<vi>)
        n128 = property class="Str"(reference=w353) -> ("Value"=w352:string)  [unwired: 1 in, 2 out]
        n129 = Build Path(base path=w341, name or relative path="Package") -> (appended path=w342:path)
        n130 = Build Path(base path=w342, name or relative path=w352) -> (appended path=w351:path)
        n131 = property on="CamSelect" class="Ring (strict)"() -> ("RingText.Text"=w345:string)  [unwired: 2 in, 2 out]
        n132 = Build Path(base path=w351, name or relative path="Vision") -> (appended path=w349:path)
        n133 = Concatenate Strings(w345, "CalTemp.png" ("name or relative path")) -> (w344:string)
        n134 = Build Path(base path=w349, name or relative path=w344) -> (appended path=w365:path)
        n135 = call "IMAQ Create"("Image Name"=w344) -> ("New Image"=w343:T1)  [unwired: 4 in, 1 out]
        n136 = local read "CalTemp"() -> (w339:T1)
        n137 = case shown="False" w358 {
          tunnel: w367 -> [w385 w386]
          tunnel: [w375 w386] -> w356
          tunnel: w366 -> [w383 _]
          tunnel: w365 -> [w382 _]
          tunnel: w343 -> [w374 _]
          tunnel: w339 -> [w371 _]
          frame False {
            w384 = "Calibration" ("Image Name")
            n138 = call "IMAQ Histogram"("error in (no error)"=w385, "Image"=w384) -> ("error out"=w379:errorcluster, "Histogram Report"=w380:T20)  [unwired: 8 in]
            n139 = call "IMAQ Equalize"("Range"=cluster{"Minimum":sgl, "Maximum":sgl} {"Minimum"=0.0, "Maximum"=255.0}, "Histogram Report"=w380, "error in (no error)"=w379, "Image Dst"=w383, "Image Src"=w384) -> ("error out"=w378:errorcluster)  [unwired: 5 in, 1 out]
            n140 = call "IMAQ Write Image And Vision Info File 2"("error in (no error)"=w378, "File Path"=w382, "Image"=w371) -> ("error out"=w376:errorcluster, "Image Out (duplicate)"=w377:T1)  [unwired: 7 in]
            n141 = call "IMAQ Copy"("error in (no error)"=w376, "Image Dst"=w374, "Image Src"=w377) -> ("error out"=w375:errorcluster, "Image Dst Out"=w373:T1)  [unwired: 3 in]
            n142 = call "IMAQ Get Calibration Info 3"("Calibration Template Image"=w373) -> ("Grid Descriptor"=→"Grid Descriptor 2":T2)  [unwired: 6 in, 8 out]
          }
          frame True {
          }
        }
        n143 = call "[FGV]Parameters.vi"(7:"Parameter"=Parameter."Write" ("Parameter"), "ParamName"="CalFilePath", 11:"Parameter"=w344) -> ("Error Out"=w364:errorcluster)  [unwired: 7 in, 1 out]
        n144 = call "[FGV]Parameters.vi"(7:"Parameter"=Parameter."Write" ("Parameter"), "Error In"=w364, "ParamName"="Cal?", 11:"Parameter"=w359) -> ("Error Out"=w346:errorcluster)  [unwired: 6 in, 1 out]
        n145 = Enqueue Element(queue=w354, element=cluster{"Message":string, "Data":variant} {"Message"="Exit", "Data"=variant}, error in (no error)=w356) -> (error out=w355:errorcluster)  [unwired: 1 in, 2 out]
        n146 = call "[FGV]Parameters.vi"("Parameter"=Parameter."Save", "Error In"=w346) -> ()  [unwired: 8 in, 2 out]
      }
      frame "Exit" {
        n147 = Release Queue(queue=w393, error in (no error)=w392) -> (error out=w388:errorcluster)  [unwired: 1 in, 2 out]
        n148 = local write "CalTemp"(w387) -> ()
      }
    }
    "Calibration Done" <- w69
    "error out" <- w64
  }
  n149 = for {
    tunnel: w7 -> [w398]
    tunnel: string[] ["Calibration", "New Image", "Select"] -> [w397] mode=indexing
    n150 = call "IMAQ Dispose"("Image"=w397, "error in (no error)"=w398) -> ()  [unwired: 4 in, 1 out]
  }
